vi "Blink LED.vi"   [LabVIEW 2015]
uses:
  Global Data.vi
  <vilib>/NI_Real-Time Target Support.lvlib
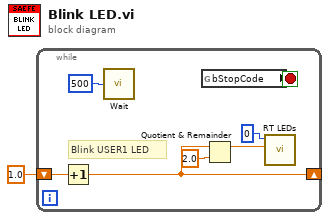
[diagram p0: block diagram]
diagram:
  n1 = while {
    shift-right: [w3] -> _
    shift-left: 1.0 ("x") -> [w7]
    stop <- w2 stop-if-true
    # "Blink USER1 LED"
    n2 = Increment(x=w7) -> (x+1=w3:dbl)
    n3 = call "Wait"("Count(mSec)"=u32 500) -> ()  [unwired: 1 out]
    n4 = global read "Global Data.vi" "bStopCode"() -> (w2:bool)
    n5 = Quotient & Remainder(x=w3, y=2.0) -> (x-y*floor(x/y)=w5:dbl)  [unwired: 1 out]
    n6 = call <vilib>:"RT LEDs.vi"("State"=w5, "LED Num"=0) -> ()  [unwired: 4 in, 2 out]
  }
